vi "AcquireSingals.vi"(6 "Funk_pom":enum32{"F:1", "F:2"}(radio), 8 "error in (no error)":errorcluster, 9 "Stop Button":bool, 10 "Num of samp":i32=1000, 11 "rate [Hz]":dbl=2000.0) -> (0 "error out":errorcluster, 1 "stopped":bool, 2 "Waveform Chart":dynamicdata(graph))   [LabVIEW 2021]
panel:
  # "Funkcje pomiarowe"
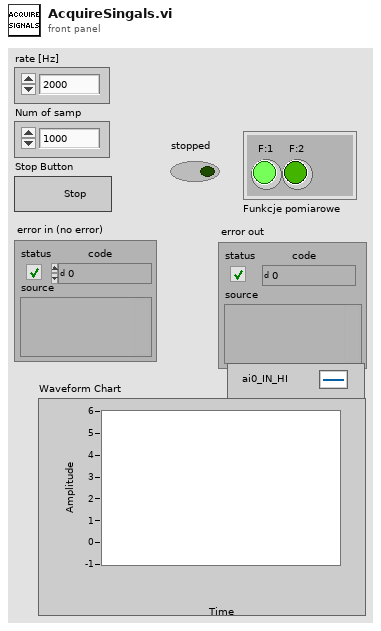
[diagram p1: front panel]
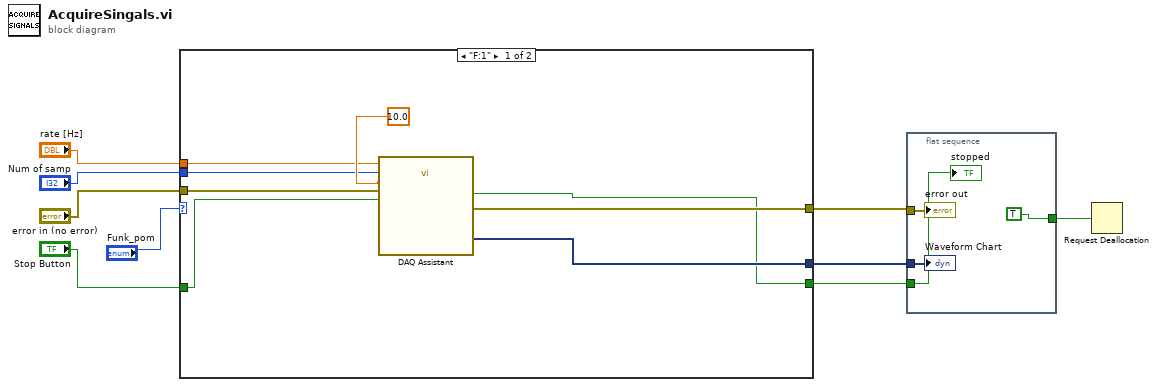
[diagram p0: block diagram]
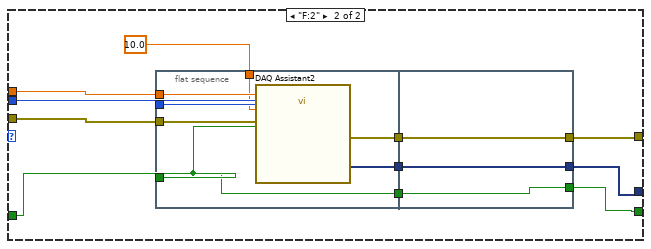
[diagram p2: hidden frame]
diagram:
  n1 = case shown="\"F:1\"" "Funk_pom" {
    tunnel: "error in (no error)" -> [w16 w25]
    tunnel: "Stop Button" -> [w11 w24]
    tunnel: "Num of samp" -> [w15 w27]
    tunnel: "rate [Hz]" -> [w14 w28]
    tunnel: [w13 w18] -> w3
    tunnel: [w12 w19] -> w2
    tunnel: [w10 w20] -> w1
    frame "F:1" {
      n2 = call "DAQ Assistant"("rate"=w14, "number of samples"=w15, "timeout (s)"=10.0, "error in"=w16, "stop (F)"=w11) -> ("data"=w12:dynamicdata, "stopped"=w10:bool, "error out"=w13:errorcluster)  [unwired: 11 in, 1 out]
    }
    frame "F:2" {
      n3 = flat-sequence {
        tunnel: w28 -> [w35]
        tunnel: w27 -> [w34]
        tunnel: 10.0 -> [w33]
        tunnel: w25 -> [w32]
        tunnel: w24 -> [w29]
        tunnel: [w31] -> w23
        tunnel: [w30] -> w22
        tunnel: [w29] -> w21
        tunnel: w23 -> [w36]
        tunnel: w22 -> [w37]
        tunnel: w21 -> [w38]
        tunnel: [w38] -> w20
        tunnel: [w37] -> w19
        tunnel: [w36] -> w18
        frame #0 {
          n4 = call "DAQ Assistant2"("rate"=w35, "number of samples"=w34, "timeout (s)"=w33, "error in"=w32, "stop (T)"=w29) -> ("data"=w30:dynamicdata, "error out"=w31:errorcluster)  [unwired: 12 in, 1 out]
        }
        frame #1 {
        }
      }
    }
  }
  n5 = flat-sequence {
    tunnel: w3 -> [w42]
    tunnel: w2 -> [w41]
    tunnel: [TRUE] -> w4
    tunnel: w1 -> [w39]
    frame #0 {
      "error out" <- w42
      "stopped" <- w39
      "Waveform Chart" <- w41
    }
  }
  n6 = Request Deallocation(w4) -> ()
